vi "Process.vi"(8 "error in":errorcluster, 11 "DAQ":refnum<class "DAQ.lvclass">) -> (0 "error out":errorcluster, 3 "DAQ out":refnum<class "DAQ.lvclass">)   [LabVIEW 2016, in "DAQ.lvclass"]
doc: "---------------------------------------------------------------\nJKI State Machine Objects™\nhttp://jki.net/state-machine-objects/\nCopyright (C) 2005-2015, JKI <info@jki.net>\nALL RIGHTS RESERVED"
uses:
  DAQ.lvclass
  C:/Program Files (x86)/National Instruments/LabVIEW 2016/vi.lib/JKI/JKI SMO/SMO/SMO.lvclass
  <vilib>/JKI/JKI SMO/SMO/Typedefs/Parent Call--Enum.ctl
  <vilib>/JKI/JKI SMO/SMO/SMO.lvclass
panel:
  out "AO.Channels":string
  out "AI.Channels":string
  # "For instructions on how to use the JKI State Machine Objects, examples and video tutorials, visit:\nhttp://jki.net/state-machine-objects/\n\nJKI State Machine Objects™\nhttp://jki.net/state-machine-objects/\nCopyright (C) 2005-2015, JKI <info@jki.net>\nALL RIGHTS RESERVED"
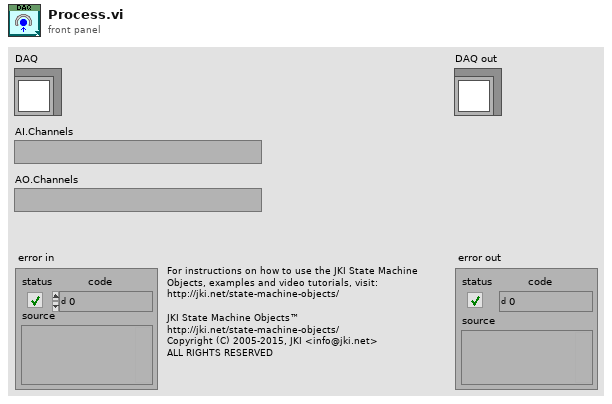
[diagram p1: front panel]
types:
  T1 = typedef "SMO.lvclass/Parent Call--Enum.ctl" = enum16{"Allows parent to run", "Does not request parent to run"}
  T2 = enum32{"invalid app kind", "Development System", "Run Time System", "Student Edition", "Embedded LabVIEW", "Evaluation", "Custom"}
  T3 = enum32{"Invalid", "Standard", "Closed", "Hidden", "Minimized", "Maximized"}
  T4 = enum32{"Bad", "Idle", "Run top level", "Running"}
  T5 = typedef "DAQ.lvclass/PrivateEvents--DAQ.AI.Channels.ctl" = string
  T6 = cluster{"Core":cluster{"Current VI Reference":refnum<vi>, "Close Panel on Exit?":bool, "error":errorcluster}, "Self Reference":refnum<class "DAQ.lvclass">, "AI.Channels":string, "AO.Channels":string}
  T7 = typedef "DAQ.lvclass/PrivateEvents--DAQ.AO.Channels.ctl" = string
  T8 = cluster{"Current VI Reference":refnum<vi>, "Close Panel on Exit?":bool, "error":errorcluster}
  T9 = typedef "SMO.lvclass/Protected Events.ctl" = cluster{"StopProcesses":refnum<user-event>, "AbortProcesses":refnum<user-event>, "Config Changed":refnum<user-event>, "Dependency":refnum<user-event>}
  T10 = typedef "DAQ.lvclass/PrivateEvents--Cluster.ctl" = cluster{"AI.Channels":refnum<user-event>, "AO.Channels":refnum<user-event>}
  T11 = typedef "DAQ.lvclass/PublicEvents--DAQ.Read.ctl" = waveform(dbl)[]
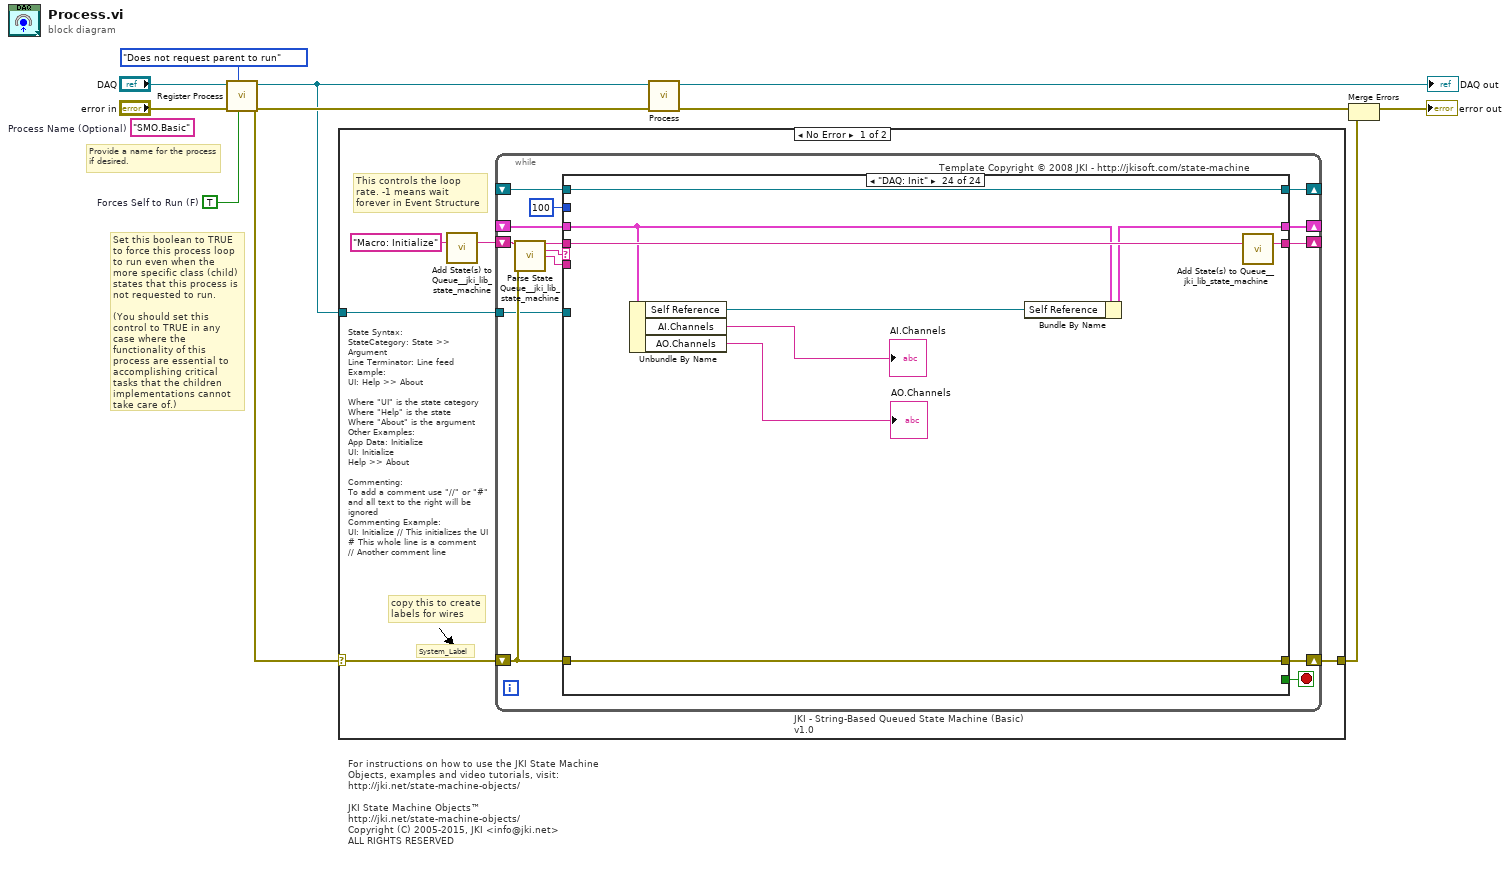
[diagram p0: block diagram]
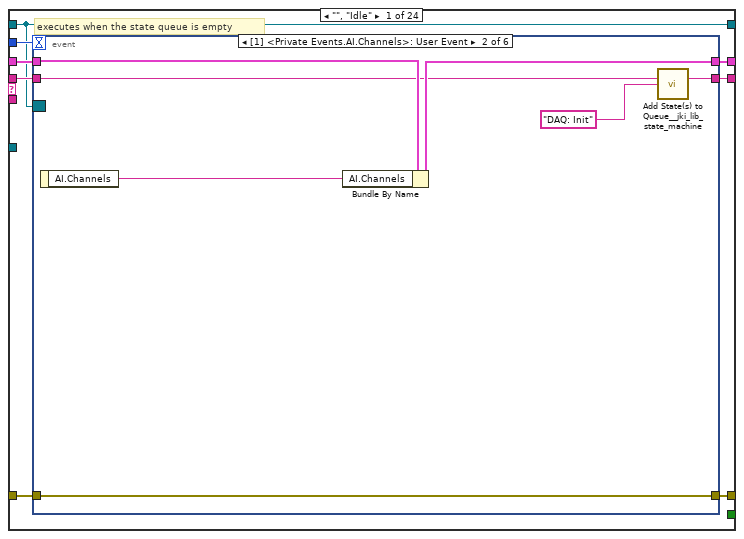
[diagram p2: hidden frame]
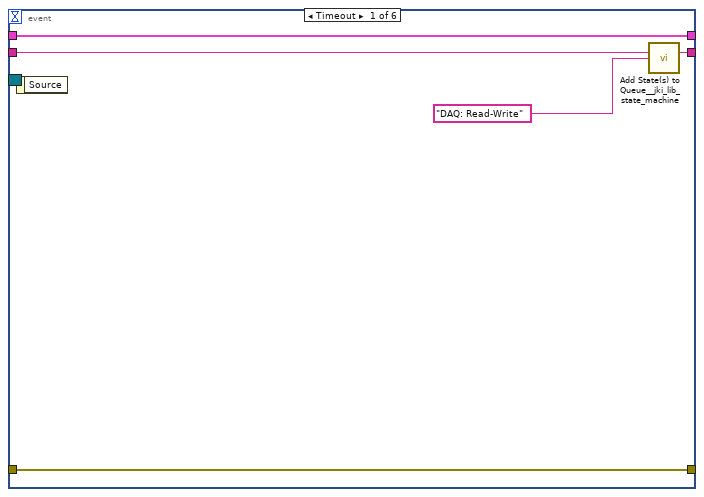
[diagram p3: hidden frame]
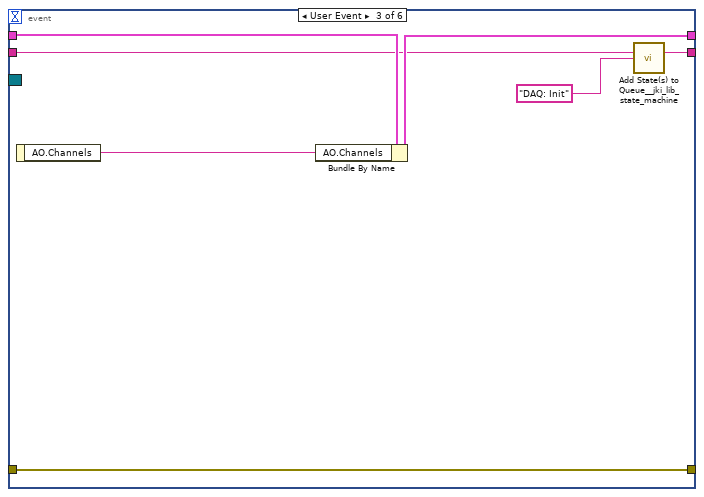
[diagram p4: hidden frame]
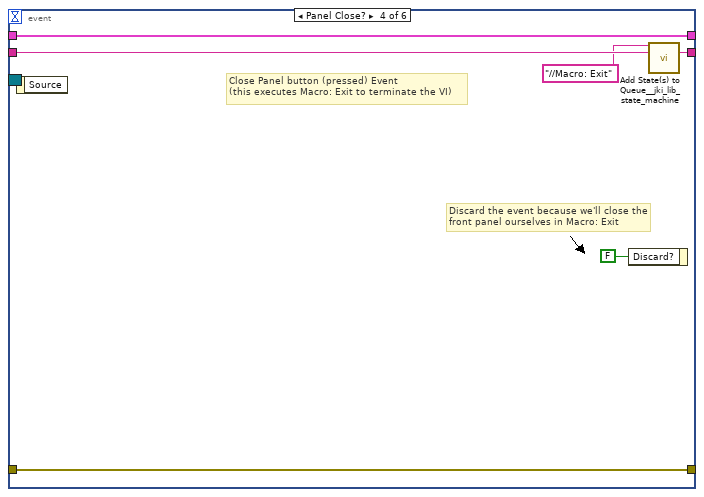
[diagram p5: hidden frame]
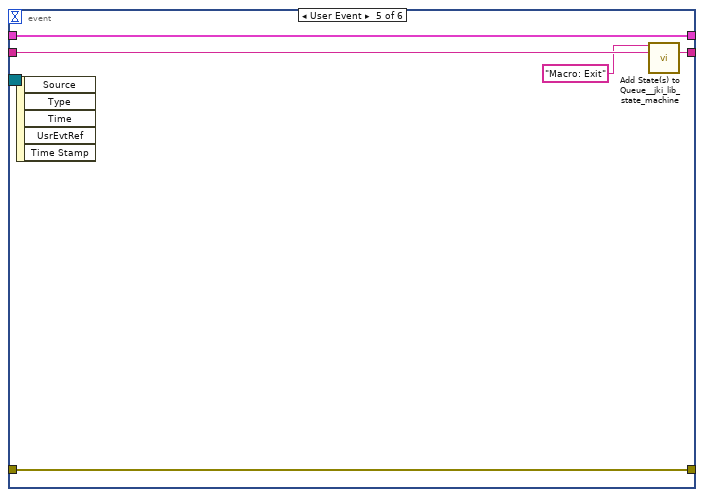
[diagram p6: hidden frame]
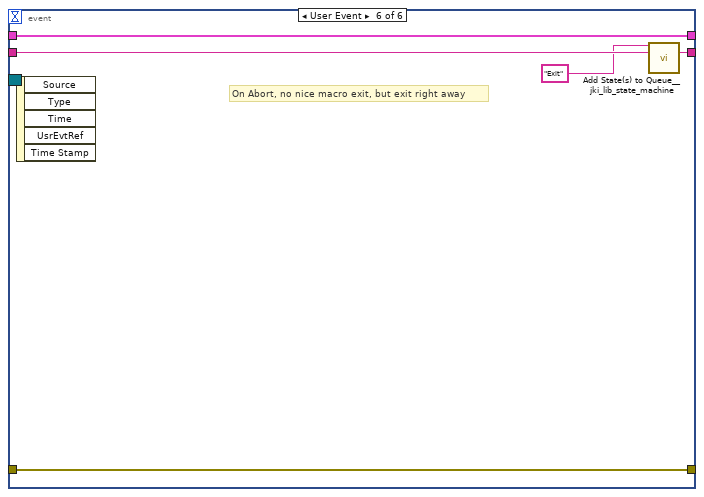
[diagram p7: hidden frame]
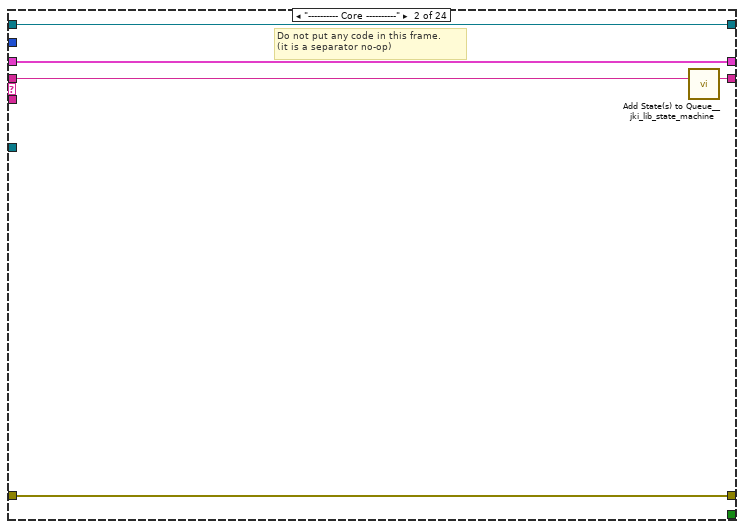
[diagram p8: hidden frame]
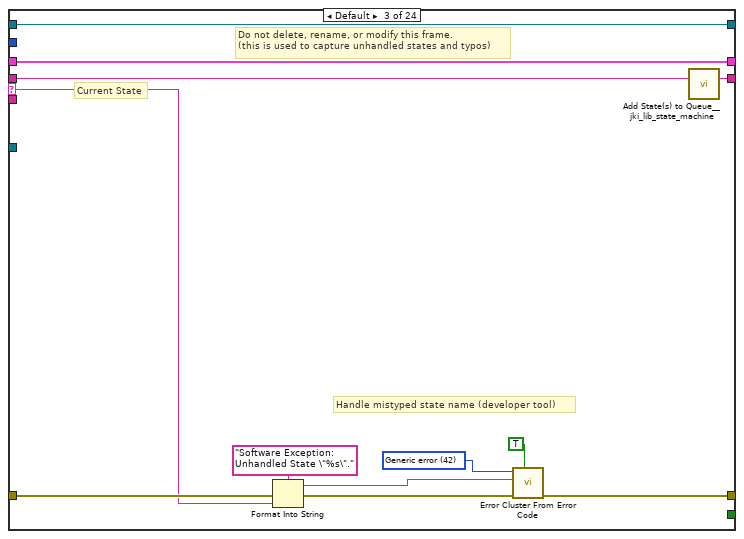
[diagram p9: hidden frame]
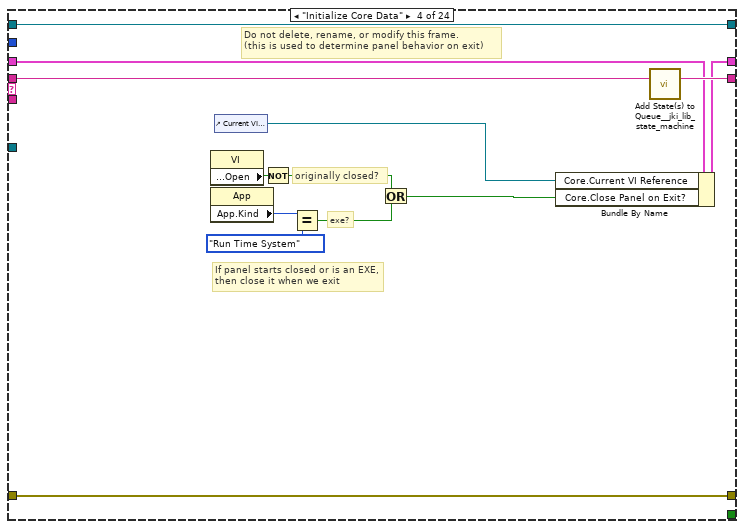
[diagram p10: hidden frame]
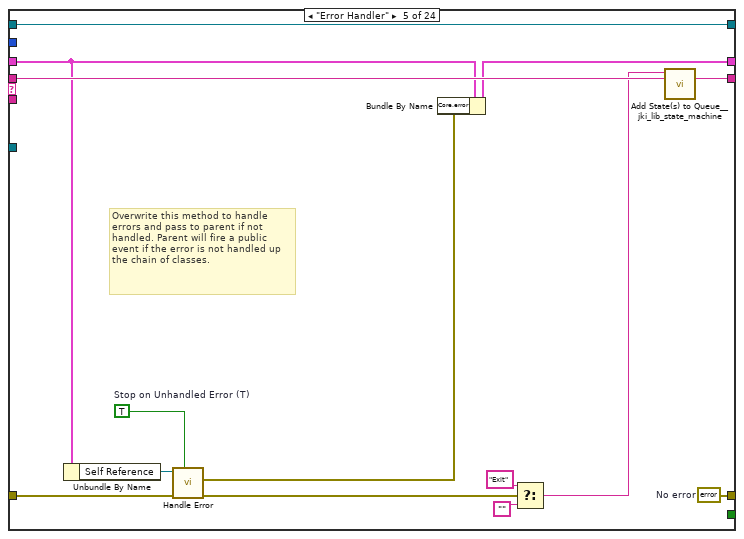
[diagram p11: hidden frame]
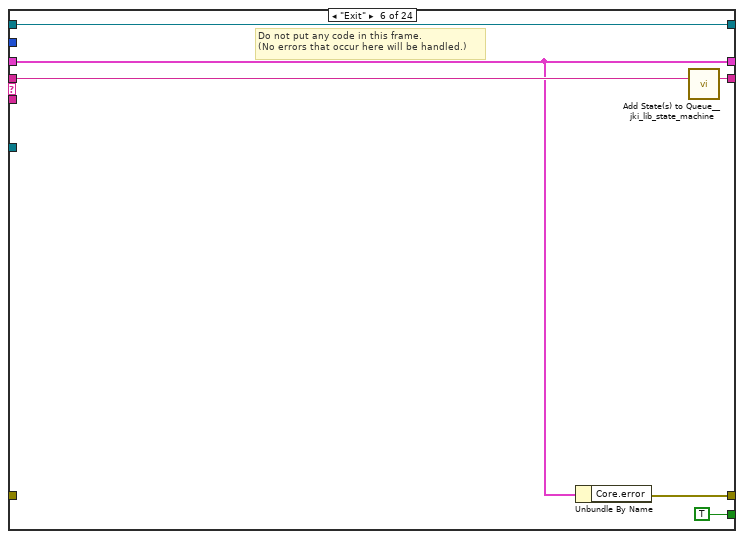
[diagram p12: hidden frame]
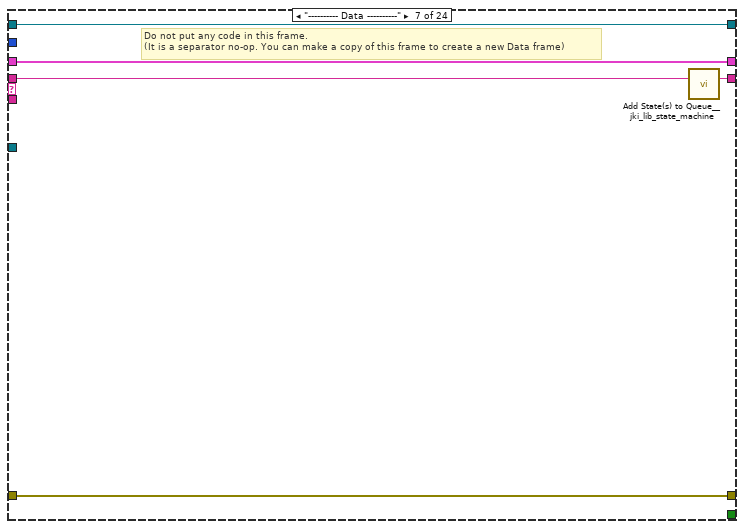
[diagram p13: hidden frame]
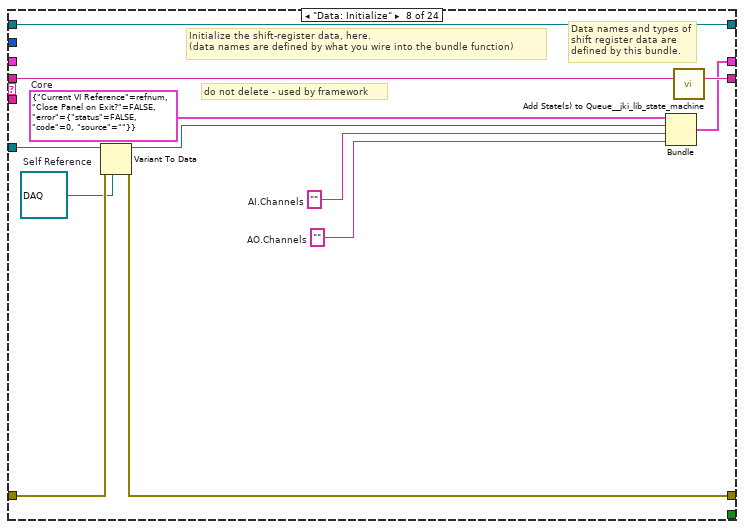
[diagram p14: hidden frame]
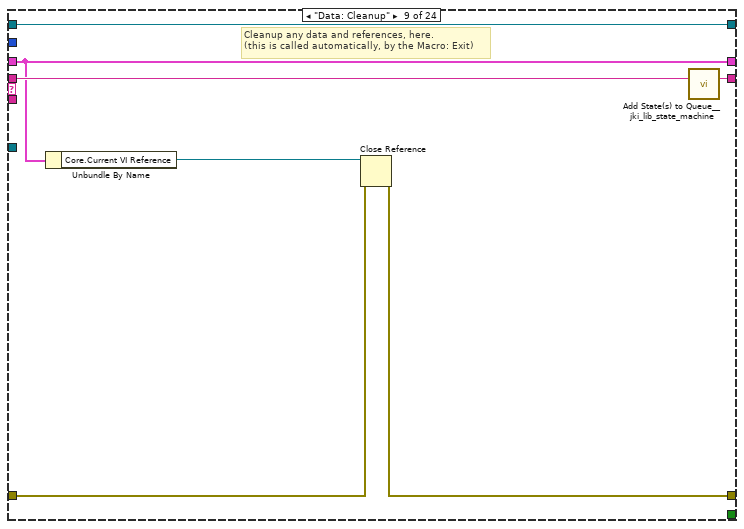
[diagram p15: hidden frame]
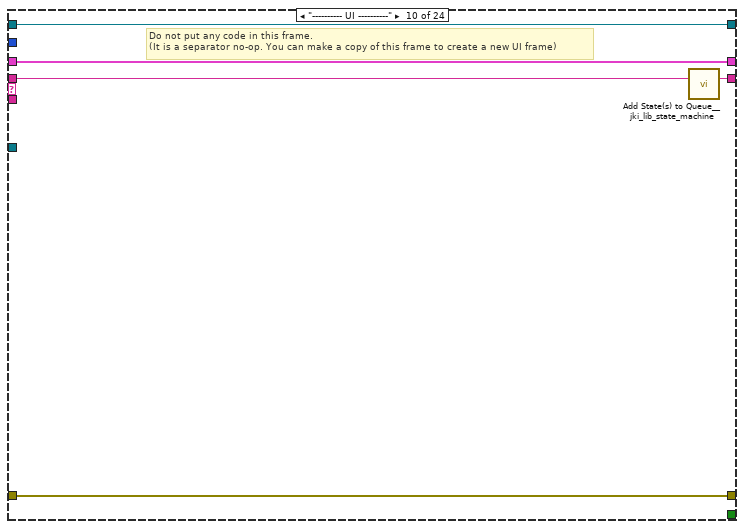
[diagram p16: hidden frame]
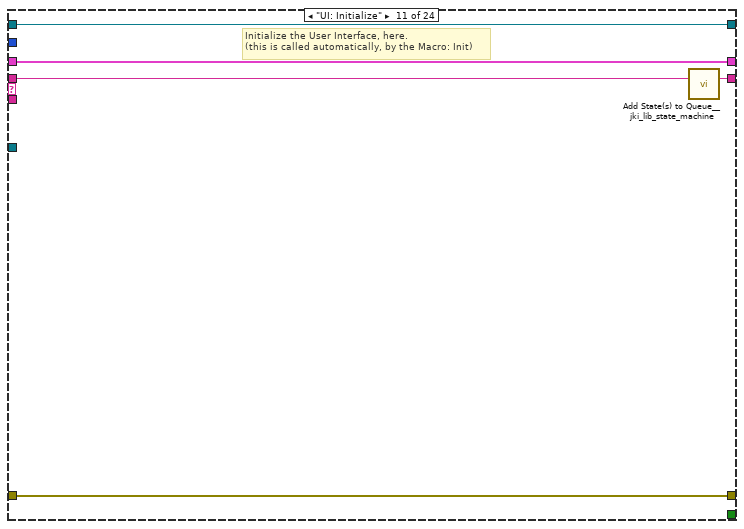
[diagram p17: hidden frame]
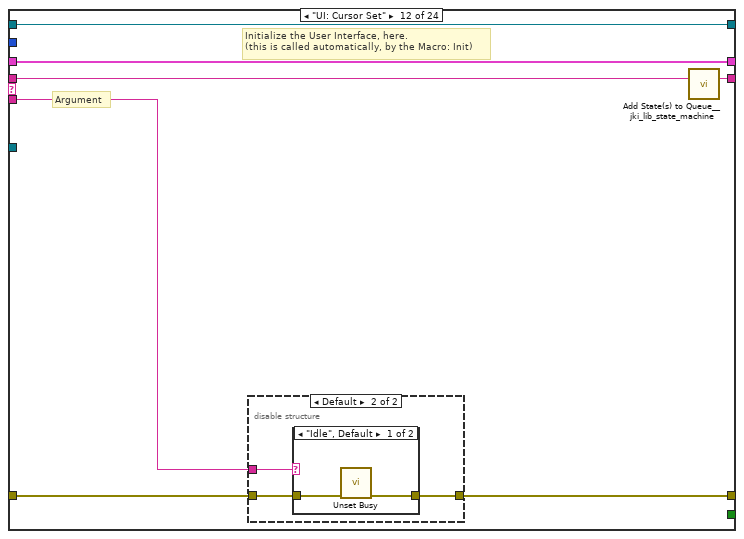
[diagram p18: hidden frame]
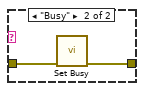
[diagram p20: hidden frame]
diagram:
  w1 = TRUE  # Forces Self to Run (F)
  (unwired) "SMO.Basic"  # Process Name (Optional)
  # "Provide a name for the process\nif desired."
  # "Set this boolean to TRUE to force this process loop to run even when the more specific class (child) states that this process is not requested to run.\n\n(You should set this control to TRUE in any case where the functionality of this process are essential to accomplishing critical tasks that the children implementations cannot take care of.)"
  # "For instructions on how to use the JKI State Machine Objects, examples and video tutorials, visit:\nhttp://jki.net/state-machine-objects/\n\nJKI State Machine Objects™\nhttp://jki.net/state-machine-objects/\nCopyright (C) 2005-2015, JKI <info@jki.net>\nALL RIGHTS RESERVED"
  n1 = call <vilib>:"Register Process.vi"("Forces Self to Run (F)"=w1, "Parent Call"=Parent_Call--Enum."Does not request parent to run", "error in (no error)"="error in", "SMO"="DAQ") -> ("error out"=w7:errorcluster, "SMO out"=w6:refnum<class "DAQ.lvclass">)  [unwired: 6 in]
  n2 = case shown="No Error" w7 {
    selector: w7 -> [w12 w306]
    tunnel: w6 -> [w13 _]
    tunnel: [w11 w306] -> w3
    frame No Error {
      # "State Syntax:\nStateCategory: State >> Argument\nLine Terminator: Line feed\nExample:\nUI: Help >> About\n\nWhere \"UI\" is the state category\nWhere \"Help\" is the state\nWhere \"About\" is the argument\nOther Examples:\nApp Data: Initialize\nUI: Initialize\nHelp >> About\n\nCommenting:\nTo add a comment use \"//\" or \"#\" and all text to the right will be ignored\nCommenting Example:\nUI: Initialize // This initializes the UI\n# This whole line is a comment\n// Another comment line"
      # "copy this to create labels for wires"
      # "This controls the loop rate. -1 means wait forever in Event Structure"
      # "System_Label"
      n3 = call <vilib>:"Add State(s) to Queue__jki_lib_state_machine.vi"("State(s) in (\"\")"="Macro: Initialize") -> ("States Out"=w15:string)  [unwired: 14 in]
      n4 = while "JKI - String-Based Queued State Machine (Basic) v1.0" {
        shift-right: [w23] -> _
        shift-left: _ -> [w22]
        shift-right: [w16] -> w11
        shift-left: w12 -> [w20]
        shift-right: [w25] -> _
        shift-left: w15 -> [w26]
        tunnel: w13 -> [w19]
        shift-right: [w18] -> _
        shift-left: _ -> [w17]
        stop <- w24 stop-if-true
        # "Template Copyright © 2008 JKI - http://jkisoft.com/state-machine"
        n5 = call <vilib>:"Parse State Queue__jki_lib_state_machine.vi"("State Queue"=w26, "Error In (no error)"=w20) -> ("Remaining States"=w28:string, "Current State"=w29:string, "Arguments"=w27:string)  [unwired: 11 in]
        n6 = case shown="\"DAQ: Init\"" w29 {
          selector: w29 -> [_ _ w79 _ _ _ _ _ _ _ _ _ _ _ _ _ _ _ _ _ _ _ _ _]
          tunnel: w28 -> [w37 w77 w83 w102 w116 w122 w127 w139 w146 w151 w156 w163 w179 w211 w225 w239 w244 w255 w260 w273 w279 w284 w296 w305]
          tunnel: w27 -> [_ _ _ _ _ _ _ _ _ _ _ w157 w173 _ _ _ _ _ _ _ _ _ _ _]
          tunnel: w22 -> [w35 w74 w81 w93 w110 w118 w124 _ w141 w148 w154 w161 w175 w208 w221 w230 w241 w252 w257 w271 w277 w282 w293 w302]
          tunnel: w20 -> [w33 w75 w84 w99 w112 _ w125 w135 w143 w149 w153 w159 w177 w209 w223 w237 w242 w247 w258 w267 w275 w280 w287 w299]
          tunnel: [w36 w76 w82 w101 w115 w121 w126 w138 w145 w150 w155 w162 w178 w210 w224 w238 w243 w254 w259 w272 w278 w283 w295 w304] -> w25
          tunnel: [_ _ _ _ _ TRUE _ _ _ _ _ _ _ _ _ _ _ _ _ _ _ _ _ _] -> w24
          tunnel: [w32 w74 w81 w100 w109 w118 w124 w137 w141 w148 w154 w161 w175 w208 w221 w230 w241 w252 w257 w271 w277 w282 w292 w301] -> w23
          tunnel: 100 ("Timeout") -> [w31 _ _ _ _ _ _ _ _ _ _ _ _ _ _ _ _ _ _ _ _ _ _ _]
          tunnel: w19 -> [_ _ _ _ _ _ _ w132 _ _ _ _ _ _ _ _ _ _ _ _ _ _ _ _]
          tunnel: [w30 w73 w78 w90 w114 w119 w123 w130 w140 w147 w152 w160 w172 w207 w222 w231 w240 w253 w256 w270 w276 w281 w294 w303] -> w18
          tunnel: w17 -> [w30 w73 w78 w90 w114 w119 w123 w130 w140 w147 w152 w160 w172 w207 w222 w231 w240 w253 w256 _ w276 w281 w294 w303]
          tunnel: [w34 w75 w85 w99 w111 w117 w125 w134 w142 w149 w153 w158 w176 w209 w223 w237 w242 w246 w258 w266 w275 w280 w285 w299] -> w16
          frame "", "Idle" {
            # "executes when the state queue is empty"
            n7 = event shown="[1] <Private Events.AI.Channels>: User Event" {
              selector: w30 -> [_ _ _ _ _ _]
              dyn-events: _ -> [_ _ _ _ _ _]
              timeout: w31 -> [_ _ _ _ _ _]
              tunnel: w37 -> [w42 w44 w51 w62 w67 w72]
              tunnel: [w41 w45 w52 w61 w66 w71] -> w36
              tunnel: w35 -> [w40 w49 w56 w59 w64 w69]
              tunnel: [w39 w46 w53 w60 w65 w70] -> w34
              tunnel: w33 -> [w39 w46 w53 w60 w65 w70]
              tunnel: [w40 w47 w54 w59 w64 w69] -> w32
              event Timeout {
                n8 = event-data() -> ()  [unwired: 1 in, 1 out]
                n9 = call <vilib>:"Add State(s) to Queue__jki_lib_state_machine.vi"("State(s) in (\"\")"=w42, "State(s) at Back (\"\")"="DAQ: Read-Write" ("State(s) at Back (\"\")")) -> ("States Out"=w41:string)  [unwired: 13 in]
              }
              event User Event {
                n10 = event-data() -> ("AI.Channels"=w48:T5)  [unwired: 1 in]
                n11 = Bundle By Name(cluster=w49, "AI.Channels"=w48) -> (w47:T6)
                n12 = call <vilib>:"Add State(s) to Queue__jki_lib_state_machine.vi"("State(s) in (\"\")"=w44, "State(s) at Back (\"\")"="DAQ: Init" ("State(s) at Back (\"\")")) -> ("States Out"=w45:string)  [unwired: 13 in]
              }
              event User Event {
                n13 = event-data() -> ("AO.Channels"=w55:T7)  [unwired: 1 in]
                n14 = Bundle By Name(cluster=w56, "AO.Channels"=w55) -> (w54:T6)
                n15 = call <vilib>:"Add State(s) to Queue__jki_lib_state_machine.vi"("State(s) in (\"\")"=w51, "State(s) at Back (\"\")"="DAQ: Init" ("State(s) at Back (\"\")")) -> ("States Out"=w52:string)  [unwired: 13 in]
              }
              event Panel Close? {
                # "Discard the event because we'll close the front panel ourselves in Macro: Exit"
                # "Close Panel button (pressed) Event\n(this executes Macro: Exit to terminate the VI)"
                n16 = event-data() -> ()  [unwired: 1 in, 1 out]
                n17 = event-data("Discard?"=FALSE) -> ()  [unwired: 1 in, 1 out]
                n18 = call <vilib>:"Add State(s) to Queue__jki_lib_state_machine.vi"("State(s) in Front (\"\")"="//Macro: Exit", "State(s) in (\"\")"=w62) -> ("States Out"=w61:string)  [unwired: 13 in]
              }
              event User Event {
                n19 = event-data() -> ()  [unwired: 1 in, 5 out]
                n20 = call <vilib>:"Add State(s) to Queue__jki_lib_state_machine.vi"("State(s) in Front (\"\")"="Macro: Exit", "State(s) in (\"\")"=w67) -> ("States Out"=w66:string)  [unwired: 13 in]
              }
              event User Event {
                # "On Abort, no nice macro exit, but exit right away"
                n21 = event-data() -> ()  [unwired: 1 in, 5 out]
                n22 = call <vilib>:"Add State(s) to Queue__jki_lib_state_machine.vi"("State(s) in Front (\"\")"="Exit", "State(s) in (\"\")"=w72) -> ("States Out"=w71:string)  [unwired: 13 in]
              }
            }
          }
          frame "---------- Core ----------" {
            # "Do not put any code in this frame.\n(it is a separator no-op)"
            n23 = call <vilib>:"Add State(s) to Queue__jki_lib_state_machine.vi"("State(s) in (\"\")"=w77) -> ("States Out"=w76:string)  [unwired: 14 in]
          }
          frame Default {
            w88 = 42 items=["No error", "Argument error", "Memory is full", "Out of zone", "End of file", "File already open", "Generic file I/O error", "File not found", "File permission error", "Disk is full", "Duplicate path", "Too many files open", "System feature not enabled", "Resource file not found", "Cannot add resource", "Resource not found", "Image not found", "Image memory error", "Pen does not exist", "Config type invalid", "Config token not found", "Config parse error", "Config memory error", "Bad external code format", "Bad external code offset", "External code not present", "Null window", "Destroy window error", "Null menu", "Print aborted", "Bad print record", "Print driver error", "Windows error during printing", "Memory error during printing", "Print dialog error", "Generic print error", "Invalid device refnum", "Device not found", "Device parameter error", "Device unit error", "Cannot open device", "Device call aborted", "Generic error", "Cancelled by user", "Object ID too low", "Object ID too high", "Object not in heap", "Unknown heap", "Unknown object (invalid DefProc)", "Unknown object (DefProc not in table)", "Message out of range", "Invalid (null) method", "Unknown message", "Manager call not supported", "Bad address", "Network operation in progress", "Network operation timed out", "Connection is busy", "Network attribute not supported", "Network error", "Address in use", "System out of memory", "Connection aborted", "Connection refused", "Not connected", "Already connected", "Connection closed", "Initialization error (interapplication manager)", "Bad occurrence", "Wait on unbound occurrence handler", "Occurrence queue overflow", "Datalog type conflict", "Unused", "Unrecognized type (interapplication manager)", "Memory corrupt", "Failed to make temporary DLL", "Old CIN version", "Drag socket not found", "Failed to load drop-object", "Failed to register OLE object", "Failed to release OLE object", "Format specifier type mismatch", "Unknown format specifier", "Too few format specifiers", "Too many format specifiers", "Scan failed", "Newer CIN version", "Error converting to variant", "Runtime menu error", "Password tampered", "Variant attribute not found", "Incompatible variant data type", "Event data is not available", "Event Store is not present", "Occurrence is not found", "Event Queue is not created", "Event info is not available", "Refnum passed is NULL", "Error retrieving Class GUID", "Error retrieving CoClass GUID", "Error retrieving TypeLib GUID.", "Bad built application magic bytes.", "Specific driver is different from the specific driver associated with the Logical Name.", "There is no session opened to the class driver.", "Max Error", "MAX - Error with config objects", "MAX - Error loading configuration", "MAX - Group not supported"]
            # "Current State"
            # "Do not delete, rename, or modify this frame.\n(this is used to capture unhandled states and typos)"
            # "Handle mistyped state name (developer tool)"
            n24 = Format Into String(format string="Software Exception: Unhandled State \"%s\"." ("message"), error in=w84, w79) -> (resulting string=w87:string, error out=w86:errorcluster)  [unwired: 1 in]
            n25 = call <vilib>:"Error Cluster From Error Code.vi"("show call chain? (False)"=TRUE, "error in (no error)"=w86, "error message (\"\")"=w87, "error code (0)"=w88) -> ("error out"=w85:errorcluster)  [unwired: 5 in]
            n26 = call <vilib>:"Add State(s) to Queue__jki_lib_state_machine.vi"("State(s) in (\"\")"=w83) -> ("States Out"=w82:string)  [unwired: 14 in]
          }
          frame "Initialize Core Data" {
            # "Do not delete, rename, or modify this frame.\n(this is used to determine panel behavior on exit)"
            # "originally closed?"
            # "exe?"
            # "If panel starts closed or is an EXE, then close it when we exit"
            n27 = property class="VI"() -> ("Front Panel.Open"=w98:bool)  [unwired: 2 in, 2 out]
            n28 = property class="App"() -> ("App.Kind"=w97:T2)  [unwired: 2 in, 2 out]
            n29 = control-ref of="Current VI Reference"() -> (w91:refnum<vi>)
            n30 = Not(x=w98) -> (.not. x?=w95:bool)
            n31 = Equal?(x=w97, y=T2."Run Time System" ("Application:Kind")) -> (x = y?=w94:bool)
            n32 = Or(x=w95, y=w94) -> (x .or. y?=w92:bool)
            n33 = Bundle By Name(cluster=w93, "Core.Current VI Reference"=w91, "Core.Close Panel on Exit?"=w92) -> (w100:T6)
            n34 = call <vilib>:"Add State(s) to Queue__jki_lib_state_machine.vi"("State(s) in (\"\")"=w102) -> ("States Out"=w101:string)  [unwired: 14 in]
          }
          frame "Error Handler" {
            w103 = TRUE  # Stop on Unhandled Error (T)
            w111 = errorcluster {"status"=FALSE, "code"=0, "source"=""}  # No error
            # "Overwrite this method to handle errors and pass to parent if not handled. Parent will fire a public event if the error is not handled up the chain of classes."
            n35 = Unbundle By Name(w110) -> ("Self Reference"=w113:refnum<class "DAQ.lvclass">)
            n36 = call-dynamic "Handle Error.vi"("Stop on Unhandled Error (T)"=w103, "error in"=w112, "SMO"=w113) -> ("handling error"=w104:errorcluster, "Unhandled error"=w107:errorcluster)  [unwired: 6 in, 1 out]
            n37 = Bundle By Name(cluster=w110, "Core.error"=w107) -> (w109:T6)
            n38 = Select(t="Exit", s=w104, f="") -> (s? t:f=w108:string)
            n39 = call <vilib>:"Add State(s) to Queue__jki_lib_state_machine.vi"("State(s) in Front (\"\")"=w108, "State(s) in (\"\")"=w116) -> ("States Out"=w115:string)  [unwired: 13 in]
          }
          frame "Exit" {
            # "Do not put any code in this frame.\n(No errors that occur here will be handled.)"
            n40 = Unbundle By Name(w118) -> ("Core.error"=w117:errorcluster)
            n41 = call <vilib>:"Add State(s) to Queue__jki_lib_state_machine.vi"("State(s) in (\"\")"=w122) -> ("States Out"=w121:string)  [unwired: 14 in]
          }
          frame "---------- Data ----------" {
            # "Do not put any code in this frame.\n(It is a separator no-op. You can make a copy of this frame to create a new Data frame)"
            n42 = call <vilib>:"Add State(s) to Queue__jki_lib_state_machine.vi"("State(s) in (\"\")"=w127) -> ("States Out"=w126:string)  [unwired: 14 in]
          }
          frame "Data: Initialize" {
            w128 = ""  # AO.Channels
            w129 = T8 {"Current VI Reference"=refnum, "Close Panel on Exit?"=FALSE, "error"={"status"=FALSE, "code"=0, "source"=""}}  # Core
            w133 = refnum<class "DAQ.lvclass"> refnum  # Self Reference
            w136 = ""  # AI.Channels
            # "do not delete - used by framework"
            # "Data names and types of shift register data are defined by this bundle."
            # "Initialize the shift-register data, here.\n(data names are defined by what you wire into the bundle function)"
            n43 = Variant To Data(error in=w135, type=w133, Variant=w132) -> (data=w131:refnum<class "DAQ.lvclass">, error out=w134:errorcluster)
            n44 = Bundle("Core"=w129, "Self Reference"=w131, "AI.Channels"=w136, "AO.Channels"=w128) -> (w137:T6)  [unwired: 1 in]
            n45 = call <vilib>:"Add State(s) to Queue__jki_lib_state_machine.vi"("State(s) in (\"\")"=w139) -> ("States Out"=w138:string)  [unwired: 14 in]
          }
          frame "Data: Cleanup" {
            # "Cleanup any data and references, here.\n(this is called automatically, by the Macro: Exit)"
            n46 = Unbundle By Name(w141) -> ("Core.Current VI Reference"=w144:refnum<vi>)
            n47 = Close Reference(reference=w144, error in (no error)=w143) -> (error out=w142:errorcluster)
            n48 = call <vilib>:"Add State(s) to Queue__jki_lib_state_machine.vi"("State(s) in (\"\")"=w146) -> ("States Out"=w145:string)  [unwired: 14 in]
          }
          frame "---------- UI ----------" {
            # "Do not put any code in this frame.\n(It is a separator no-op. You can make a copy of this frame to create a new UI frame)"
            n49 = call <vilib>:"Add State(s) to Queue__jki_lib_state_machine.vi"("State(s) in (\"\")"=w151) -> ("States Out"=w150:string)  [unwired: 14 in]
          }
          frame "UI: Initialize" {
            # "Initialize the User Interface, here.\n(this is called automatically, by the Macro: Init)"
            n50 = call <vilib>:"Add State(s) to Queue__jki_lib_state_machine.vi"("State(s) in (\"\")"=w156) -> ("States Out"=w155:string)  [unwired: 14 in]
          }
          frame "UI: Cursor Set" {
            # "Argument"
            # "Initialize the User Interface, here.\n(this is called automatically, by the Macro: Init)"
            n51 = disable-structure shown="Default" {
              disable-tunnel: w159 -> [w164 w167]
              disable-tunnel: [w164 w166] -> w158
              disable-tunnel: w157 -> [_ w165]
              frame condition #0 {
              }
              frame condition #1 (active) {
                n52 = case shown="\"Idle\", Default" w165 {
                  tunnel: w167 -> [w169 w171]
                  tunnel: [w168 w170] -> w166
                  frame "Idle", Default {
                    n53 = call <vilib>:"Unset Busy.vi"("error in (no error)"=w169) -> ("error out"=w168:errorcluster)  [unwired: 10 in]
                  }
                  frame "Busy" {
                    n54 = call <vilib>:"Set Busy.vi"("error in (no error)"=w171) -> ("error out"=w170:errorcluster)  [unwired: 9 in, 1 out]
                  }
                }
              }
            }
            n55 = call <vilib>:"Add State(s) to Queue__jki_lib_state_machine.vi"("State(s) in (\"\")"=w163) -> ("States Out"=w162:string)  [unwired: 14 in]
          }
          frame "UI: Front Panel State" {
            # "Argument"
            # "Set Front Panel Open or Closed\n(Usage: \"UI: Front Panel State >> Open|Close\")"
            n56 = Unbundle By Name(w175) -> ("Core.Current VI Reference"=w174:refnum<vi>)
            n57 = disable-structure shown="Default" {
              disable-tunnel: w177 -> [w183 w206]
              disable-tunnel: [w182 w206] -> w176
              disable-tunnel: w174 -> [w181 _]
              disable-tunnel: w173 -> [w180 _]
              frame condition #0 (active) {
                n58 = case shown="\"Close\"" w180 {
                  tunnel: w183 -> [w187 w200]
                  tunnel: [w189 w201] -> w182
                  tunnel: w181 -> [w188 w198]
                  frame "Open", Default {
                    n59 = property class="VI"(reference=w188, error in=w187) -> (reference out=w185:refnum<vi>, error out=w186:errorcluster, "FP.State"=w184:T3)
                    n60 = case shown="\"Closed\"" w184 {
                      tunnel: [w192 w195] -> w189
                      tunnel: w186 -> [w191 w195]
                      tunnel: w185 -> [w190 _]
                      frame "Closed" {
                        n61 = invoke class="VI" method="FP.Open"(reference=w190, error in=w191, "Activate"=TRUE, "State"=T3."Standard") -> (error out=w192:errorcluster)  [unwired: 1 in, 4 out]
                      }
                      frame Default {
                      }
                    }
                  }
                  frame "Close" {
                    n62 = property class="VI"(reference=w198, error in=w200) -> (reference out=w197:refnum<vi>, error out=w199:errorcluster, "FP.State"=w196:T3)
                    n63 = case shown="Default" w196 {
                      tunnel: [w202 w205] -> w201
                      tunnel: w199 -> [w202 w204]
                      tunnel: w197 -> [_ w203]
                      frame "Invalid", "Closed" {
                      }
                      frame Default {
                        n64 = invoke class="VI" method="FP.Close"(reference=w203, error in=w204) -> (error out=w205:errorcluster)  [unwired: 1 in, 2 out]
                      }
                    }
                  }
                }
              }
              frame condition #1 {
              }
            }
            n65 = call <vilib>:"Add State(s) to Queue__jki_lib_state_machine.vi"("State(s) in (\"\")"=w179) -> ("States Out"=w178:string)  [unwired: 14 in]
          }
          frame "---------- Macro ----------" {
            # "Do not put any code in this frame.\n(It is a separator no-op. You can make a copy of this frame to create a new Macro frame)"
            n66 = call <vilib>:"Add State(s) to Queue__jki_lib_state_machine.vi"("State(s) in (\"\")"=w211) -> ("States Out"=w210:string)  [unwired: 14 in]
          }
          frame "Macro: Initialize" {
            w216 = "UI: Initialize\nUI: Front Panel State >> Open"  # UI: Initialize UI: Front Panel State >> Open
            w212 = "Process: Sync"
            # "Initialization Macro\n(This is called once, when the VI starts)"
            n67 = control-ref of="This VI"() -> (w214:refnum<vi>)
            n68 = property class="VI"(reference=w214) -> ("Exec.State"=w213:T4)  [unwired: 1 in, 2 out]
            n69 = Equal?(x=w213, y=T4."Run top level") -> (x = y?=w219:bool)
            n70 = Select(t=w212, s=w219, f="") -> ()  [unwired: 1 out]
            n71 = call <vilib>:"Add State(s) to Queue__jki_lib_state_machine.vi"("State(s) in Front (\"\")"="Data: Initialize\nInitialize Core Data\nEvents: Register", "State(s) in (\"\")"=w212, "State(s) at Back (\"\")"=w216) -> ("States Out"=w215:string)  [unwired: 12 in]
            n72 = call <vilib>:"Add State(s) to Queue__jki_lib_state_machine.vi"("State(s) in Front (\"\")"=w215, "State(s) in (\"\")"=w225) -> ("States Out"=w224:string)  [unwired: 13 in]
          }
          frame "Macro: Exit" {
            # "Exit Macro\n(This is called once, when the VI exits)"
            n73 = Unbundle By Name(w230) -> ("Core.Close Panel on Exit?"=w236:bool)
            n74 = Select(t="UI: Front Panel State >> Close", s=w236, f="") -> (s? t:f=w233:string)
            n75 = call <vilib>:"Add State(s) to Queue__jki_lib_state_machine.vi"("State(s) in Front (\"\")"="Data: Cleanup\nEvents: Unregister", "State(s) in (\"\")"="Process: Sync", "State(s) at Back (\"\")"="Exit") -> ("States Out"=w227:string)  [unwired: 12 in]
            n76 = call <vilib>:"Add State(s) to Queue__jki_lib_state_machine.vi"("State(s) in (\"\")"=w233, "State(s) at Back (\"\")"=w227) -> ("States Out"=w232:string)  [unwired: 13 in]
            n77 = call <vilib>:"Add State(s) to Queue__jki_lib_state_machine.vi"("State(s) in Front (\"\")"=w232, "State(s) in (\"\")"=w239) -> ("States Out"=w238:string)  [unwired: 13 in]
          }
          frame "---------- Process ----------" {
            # "Template Separator\n(You can make a copy of, or modify, this frame)"
            n78 = call <vilib>:"Add State(s) to Queue__jki_lib_state_machine.vi"("State(s) in (\"\")"=w244) -> ("States Out"=w243:string)  [unwired: 14 in]
          }
          frame "Process: Sync" {
            n79 = Unbundle By Name(w252) -> ("Self Reference"=w248:refnum<class "DAQ.lvclass">)
            n80 = call <vilib>:"WaitOnProcessSync.vi"("error in (no error)"=w247, "SMO"=w248) -> ("error out"=w246:errorcluster, "Don't run?"=w251:bool)  [unwired: 7 in, 1 out]
            n81 = Select(t="Data: Cleanup\nEvents: Unregister\nExit", s=w251, f="") -> (s? t:f=w245:string)
            n82 = call <vilib>:"Add State(s) to Queue__jki_lib_state_machine.vi"("State(s) in Front (\"\")"=w245, "State(s) in (\"\")"=w255) -> ("States Out"=w254:string)  [unwired: 13 in]
          }
          frame "---------- Events ----------" {
            # "Template Separator\n(You can make a copy of, or modify, this frame)"
            n83 = call <vilib>:"Add State(s) to Queue__jki_lib_state_machine.vi"("State(s) in (\"\")"=w260) -> ("States Out"=w259:string)  [unwired: 14 in]
          }
          frame "Events: Register" {
            # "Expand to add\nmore events"
            n84 = Unbundle By Name(w271) -> ("Self Reference"=w268:refnum<class "DAQ.lvclass">)
            n85 = call <vilib>:"GetProtectedEvents.vi"("SMO"=w268) -> ("error out"=w264:errorcluster, "SMO Protected Events"=w269:T9, "SMO out"=w261:refnum<class "DAQ.lvclass">)  [unwired: 8 in]
            n86 = call "DAQ.GetPrivateEvents.vi"("DAQ"=w261) -> ("error out"=w263:errorcluster, "Private Events"=w262:T10)  [unwired: 8 in, 1 out]
            n87 = register-events(w269, w262) -> (reference out=w270:refnum<event-registration>, error out=w265:errorcluster)  [unwired: 2 in]
            n88 = Merge Errors(w267, w265, w264, w263) -> (w266:errorcluster)
            n89 = call <vilib>:"Add State(s) to Queue__jki_lib_state_machine.vi"("State(s) in (\"\")"=w273) -> ("States Out"=w272:string)  [unwired: 14 in]
          }
          frame "Events: Unregister" {
            n90 = Unregister For Events(event registration refnum=w276, error in=w275) -> (error out=w274:errorcluster)
            n91 = call <vilib>:"Clear Errors.vi"("error in (no error)"=w274) -> ()  [unwired: 5 in, 2 out]
            n92 = call <vilib>:"Add State(s) to Queue__jki_lib_state_machine.vi"("State(s) in (\"\")"=w279) -> ("States Out"=w278:string)  [unwired: 14 in]
          }
          frame "---------- Action ----------" {
            n93 = call <vilib>:"Add State(s) to Queue__jki_lib_state_machine.vi"("State(s) in (\"\")"=w284) -> ("States Out"=w283:string)  [unwired: 14 in]
          }
          frame "DAQ: Read-Write" {
            n94 = Unbundle By Name(w293) -> ("Self Reference"=w289:refnum<class "DAQ.lvclass">)
            n95 = call-dynamic "DAQ.Read.Override.vi"("error in (no error)"=w287, "DAQ in"=w289) -> ("error out"=w286:errorcluster, "Read"=w290:T11, "DAQ out"=w288:refnum<class "DAQ.lvclass">)  [unwired: 7 in]
            n96 = call "DAQ.Read.vi"("error in (no error)"=w286, "Read"=w290, "DAQ"=w288) -> ("error out"=w285:errorcluster, "DAQ out"=w291:refnum<class "DAQ.lvclass">)  [unwired: 7 in]
            n97 = Bundle By Name(cluster=w293, "Self Reference"=w291) -> (w292:T6)
            n98 = call <vilib>:"Add State(s) to Queue__jki_lib_state_machine.vi"("State(s) in (\"\")"=w296) -> ("States Out"=w295:string)  [unwired: 14 in]
          }
          frame "DAQ: Init" {
            n99 = Unbundle By Name(w302) -> ("Self Reference"=w300:refnum<class "DAQ.lvclass">, "AI.Channels"=→"AI.Channels":string, "AO.Channels"=→"AO.Channels":string)
            n100 = Bundle By Name(cluster=w302, "Self Reference"=w300) -> (w301:T6)
            n101 = call <vilib>:"Add State(s) to Queue__jki_lib_state_machine.vi"("State(s) in (\"\")"=w305) -> ("States Out"=w304:string)  [unwired: 14 in]
          }
        }
      }
    }
    frame Error {
    }
  }
  n102 = call-parent "Process.vi"("error in"=w7, "SMO"=w6) -> ("error out"=w4:errorcluster, "SMO out"=→"DAQ out":refnum<class "DAQ.lvclass">)  [unwired: 8 in]
  n103 = Merge Errors(w4, w3) -> (→"error out":errorcluster)
